vi "Reset.vi"(11 "ExpFitter in":refnum<class "ExpFitter.lvclass">) -> (3 "ExpFitter out":refnum<class "ExpFitter.lvclass">)   [LabVIEW 2019, in "ExpFitter.lvclass"]
uses:
  ExpFitter.lvclass
  ExpFitter.lvclass/ExpFitter.ctl
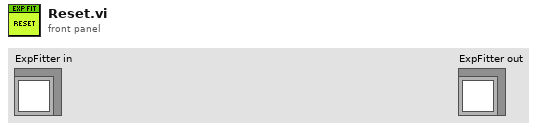
[diagram p1: front panel]
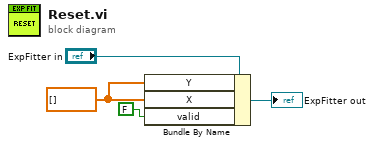
[diagram p0: block diagram]
diagram:
  w2 = dbl[] [] ("Y")
  n1 = Bundle By Name(cluster="ExpFitter in", "Y"=w2, "X"=w2, "valid"=FALSE ("DataExpFit.valid")) -> (→"ExpFitter out":refnum<class "ExpFitter.lvclass">)
